vi "Release-process-notifiers.vi"(8 "error in (no error)":errorcluster, 11 "Data ref. in":refnum<data-value>) -> (0 "error out":errorcluster, 3 "Data ref.":refnum<data-value>)   [LabVIEW 2013, in "CameraVision.lvlib" / "CV-Main.lvclass"]
uses:
  CV-Main.lvclass
  CV-Main.lvclass/CV-Main.ctl
  Read Acq stats.vi
  Read UI buffer.vi
  Read Map.vi
  Read Processing.vi
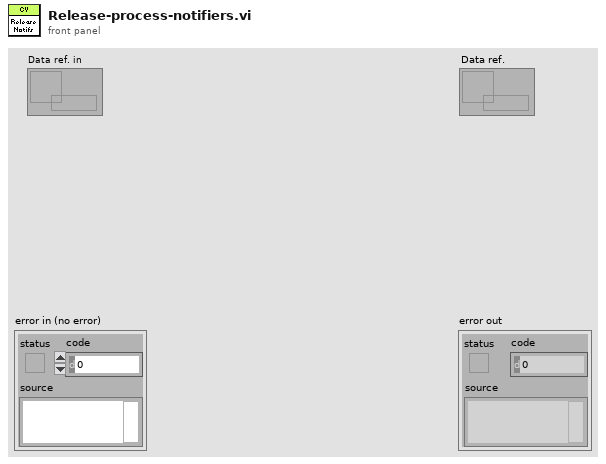
[diagram p1: front panel]
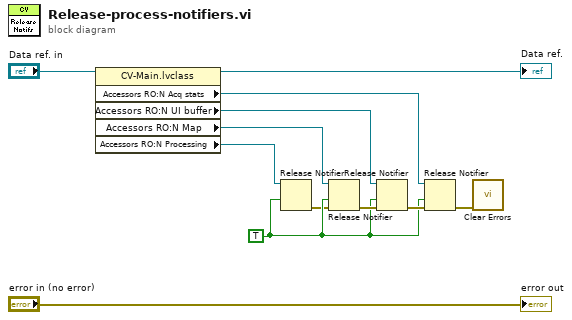
[diagram p0: block diagram]
diagram:
  w9 = TRUE ("force destroy? (F)")
  n1 = property class="CV-Main.lvclass"(reference="Data ref. in") -> (reference out=→"Data ref.":refnum<data-value>, "Accessors RO:N Acq stats"=w5:refnum<notifier>, "Accessors RO:N UI buffer"=w4:refnum<notifier>, "Accessors RO:N Map"=w3:refnum<notifier>, "Accessors RO:N Processing"=w2:refnum<notifier>)  [unwired: 1 in, 1 out]
  n2 = Release Notifier(notifier=w2, force destroy? (F)=w9) -> (error out=w1:errorcluster)  [unwired: 1 in, 2 out]
  n3 = Release Notifier(notifier=w3, force destroy? (F)=w9, error in (no error)=w1) -> (error out=w11:errorcluster)  [unwired: 2 out]
  n4 = Release Notifier(notifier=w4, force destroy? (F)=w9, error in (no error)=w11) -> (error out=w10:errorcluster)  [unwired: 2 out]
  n5 = Release Notifier(notifier=w5, force destroy? (F)=w9, error in (no error)=w10) -> (error out=w8:errorcluster)  [unwired: 2 out]
  n6 = call <vilib>:"Clear Errors.vi"("error in (no error)"=w8) -> ()  [unwired: 6 in, 1 out]
  "error out" <- "error in (no error)"
